vi "TDC_main.vi"() -> ()   [LabVIEW 2014]
panel:
  out "建过表":bool
  out "时间多道状态":string
  in  "放大":bool
  in  "复位":bool
  in  "是否需要建立修正表":bool
  out "时间谱":dbl[](array[numeric])
  out "修正后时间":dbl[](array[numeric])
  out "b查找表":dbl[](graph)
  out "a查找表":dbl[](graph)
  out "b积分表":dbl[](array[numeric])
  out "a积分表":dbl[](array[numeric])
  out "b码密度":dbl[](graph)
  out "a码密度":dbl[](graph)
  out "码密度数据量":dbl
  out "b细时间分布":dbl[](array[numeric])
  out "a细时间分布谱":dbl[](array[numeric])
  out "时间数据":u32[](array[numeric])
  out "起始时间":dbl
  in  "电压":u16=500
  in  "收发数据":T1(ring)
  out "保存灯":bool
  out "寻峰灯":bool
  out "状态灯":bool
  in  "按键检测":enum16{"空闲", "开始", "停止", "寻峰", "保存", "退出"}(ring)
  in  "保存":bool
  in  "寻峰":bool
  in  "停止":bool
  in  "开始":bool
  out "时间分布谱":dbl[](graph)
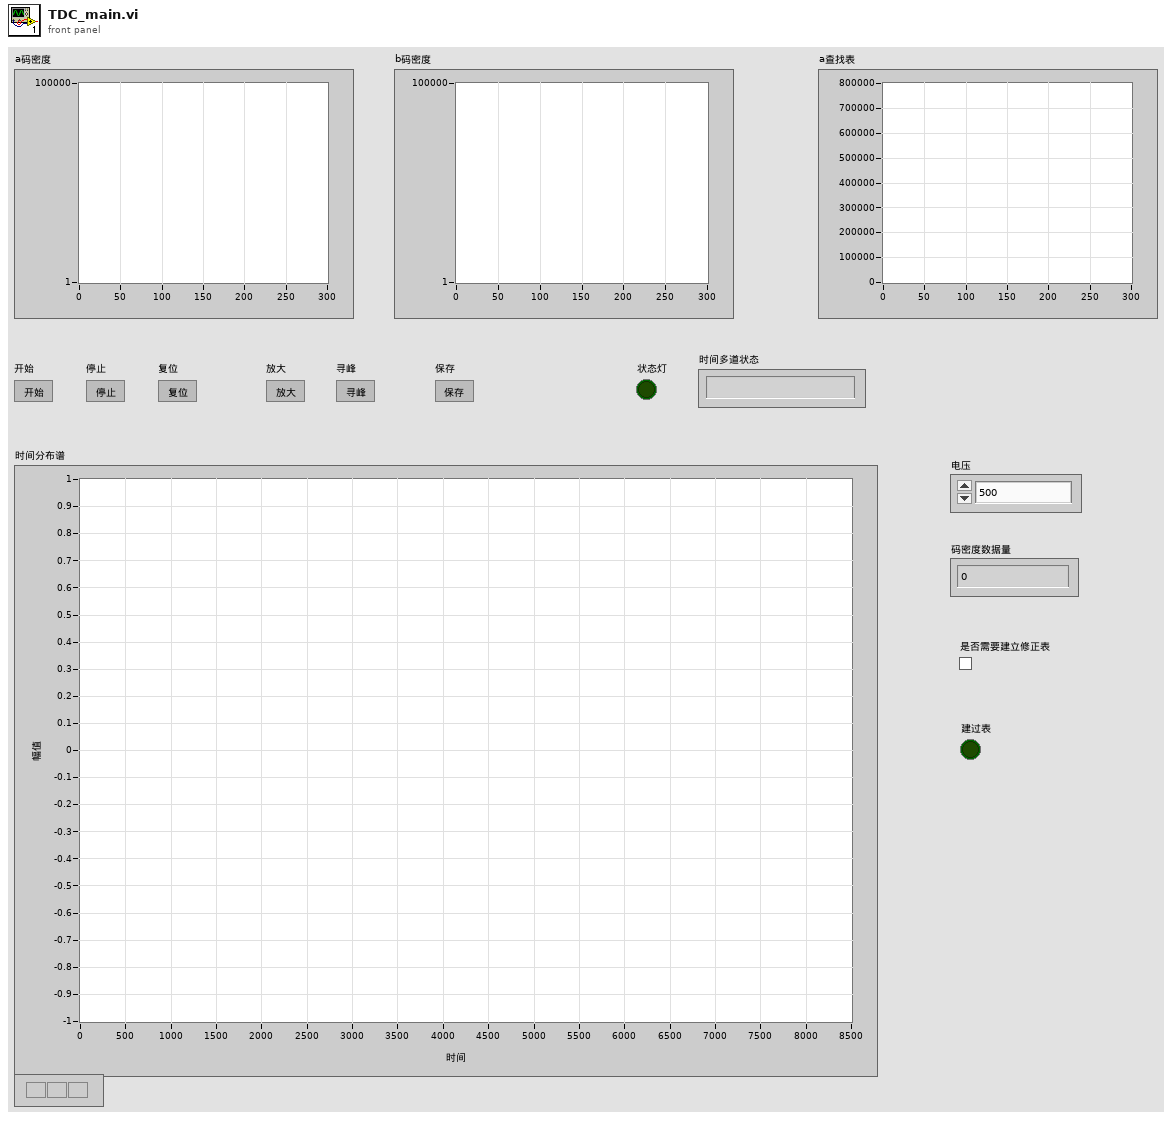
[diagram p1: front panel]
types:
  T1 = enum16{"空闲", "配置", "使能", "建立码密度表", "建立查找表", "显示时间谱"}
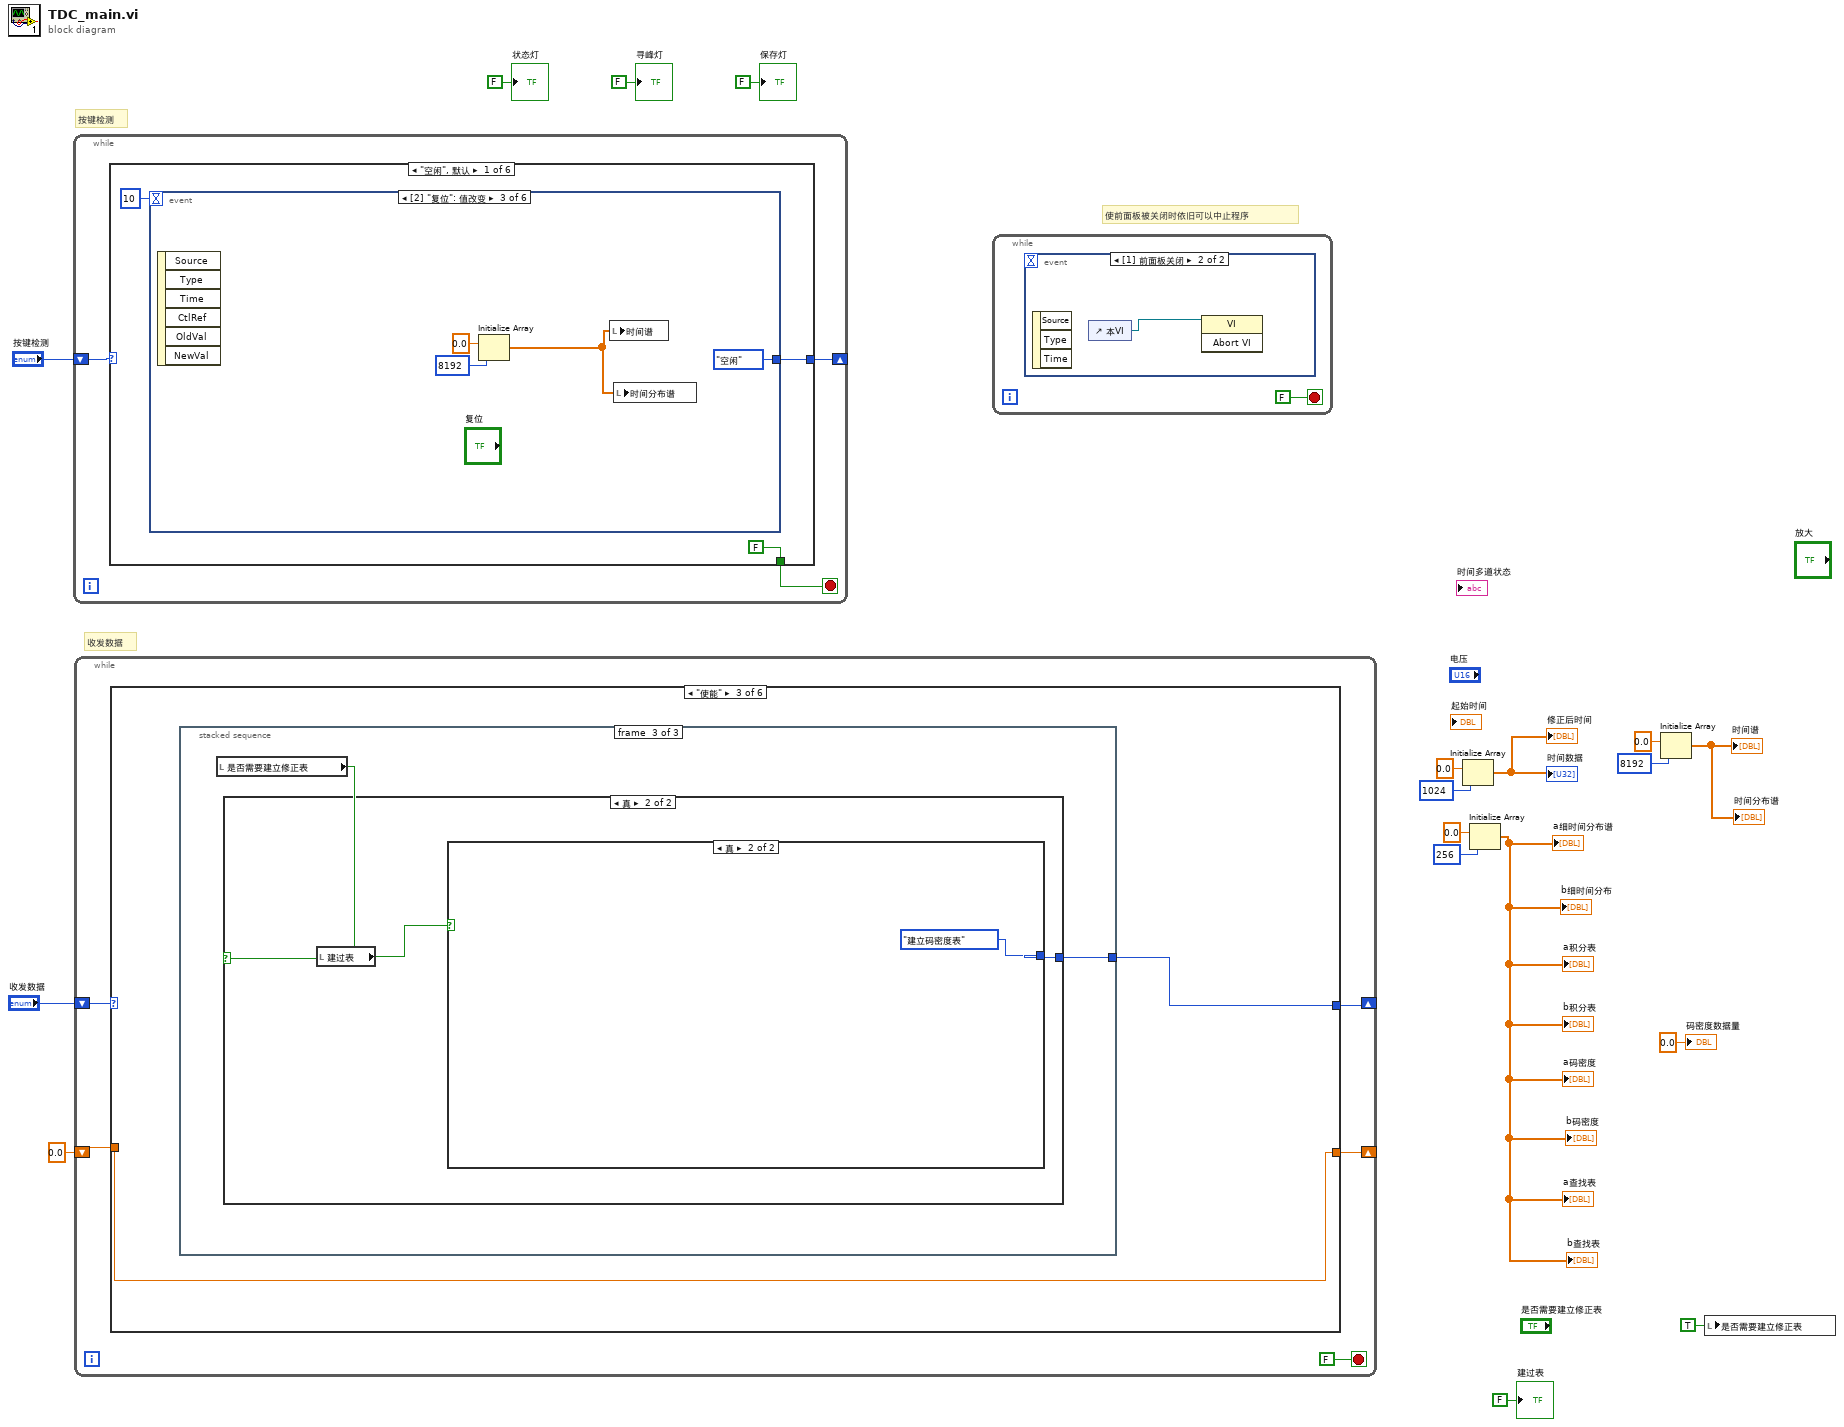
[diagram p0: block diagram]
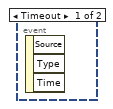
[diagram p2: hidden frame]
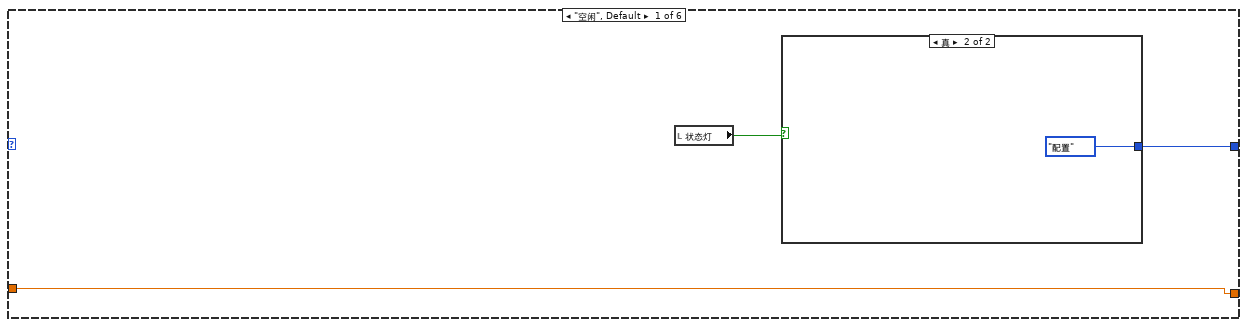
[diagram p3: hidden frame]
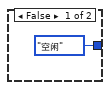
[diagram p4: hidden frame]
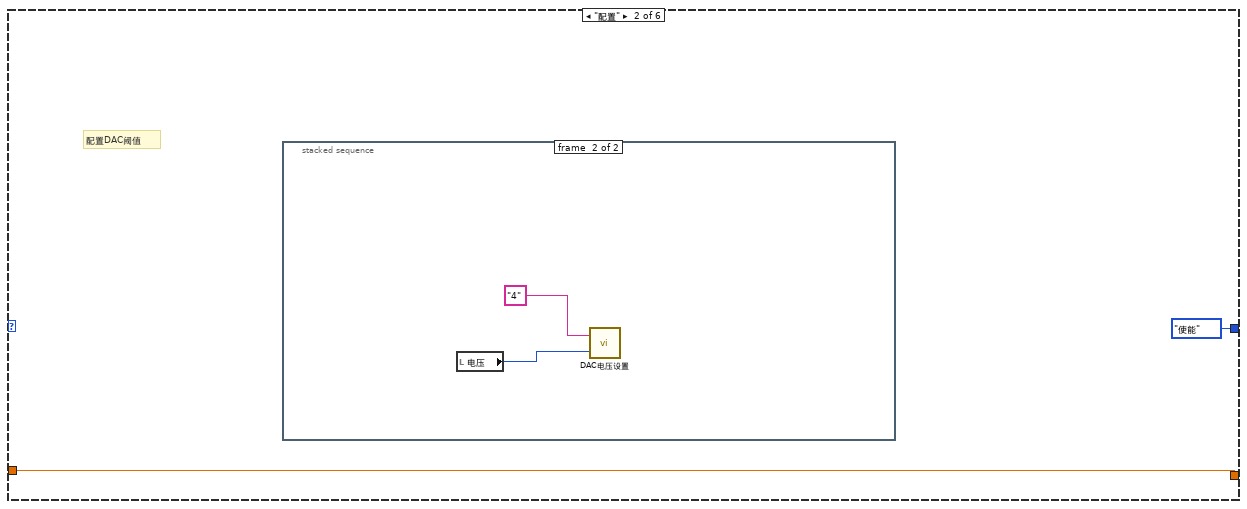
[diagram p5: hidden frame]
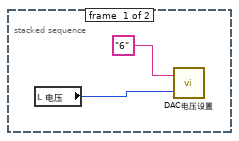
[diagram p6: hidden frame]
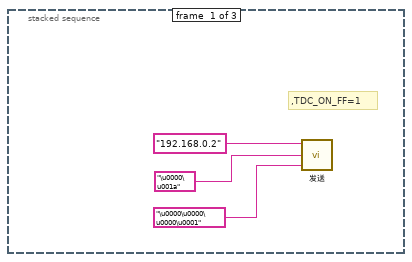
[diagram p7: hidden frame]
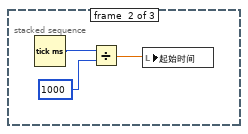
[diagram p8: hidden frame]
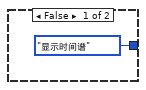
[diagram p9: hidden frame]
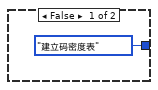
[diagram p10: hidden frame]
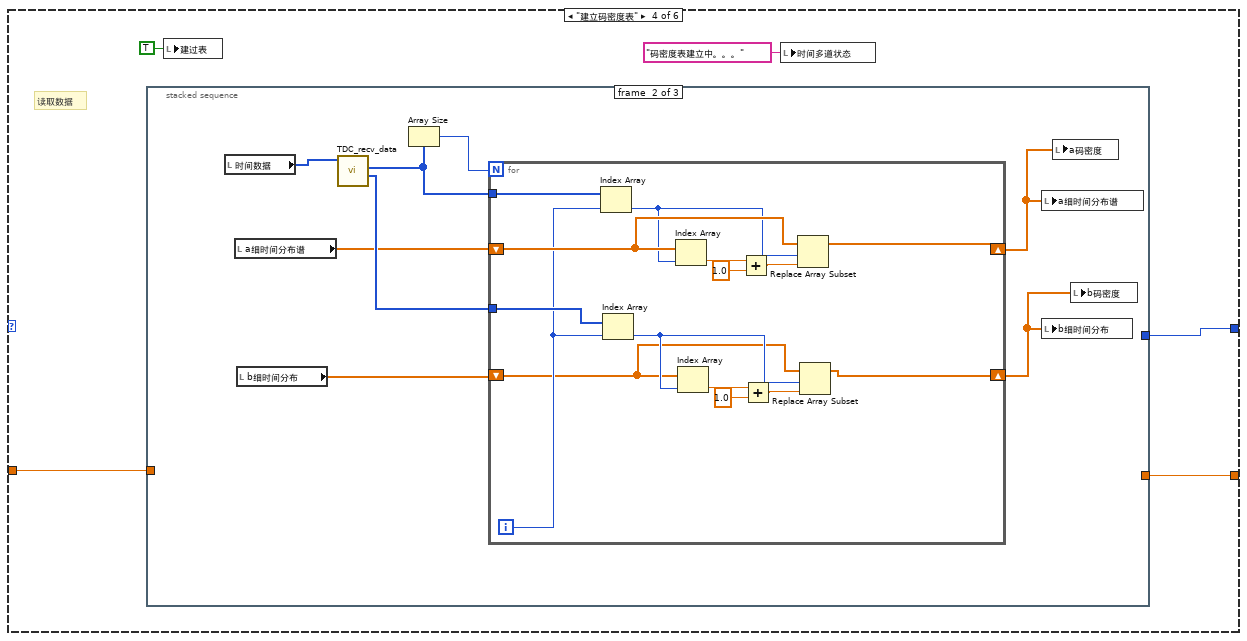
[diagram p11: hidden frame]
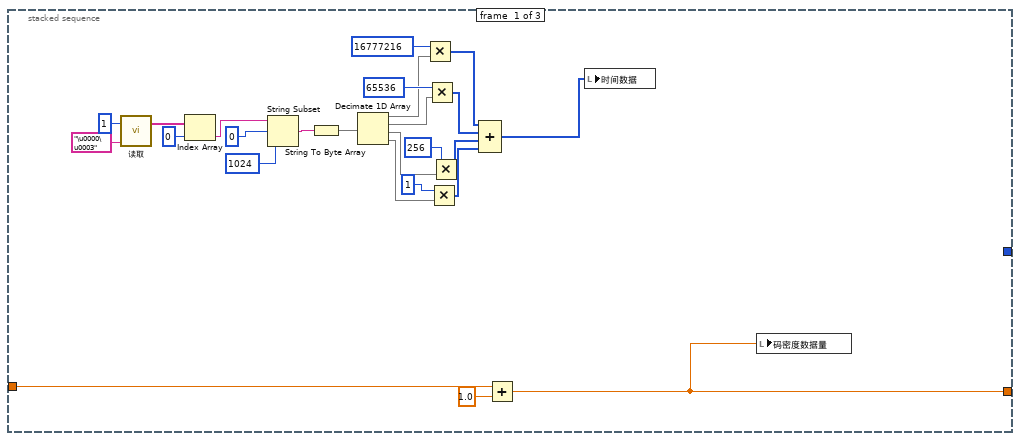
[diagram p12: hidden frame]
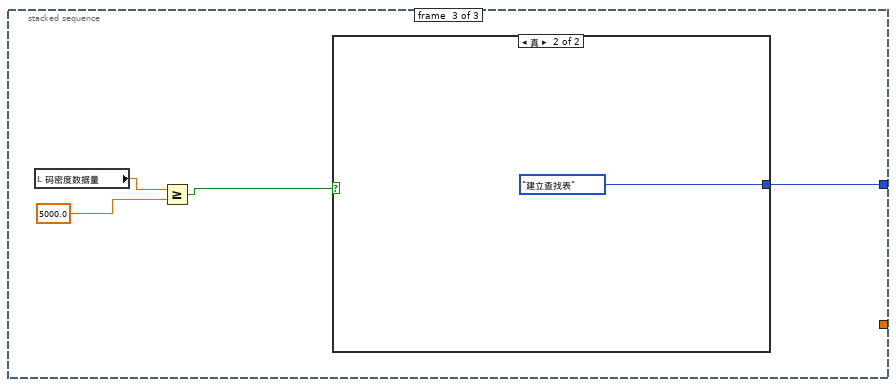
[diagram p13: hidden frame]
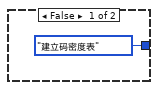
[diagram p14: hidden frame]
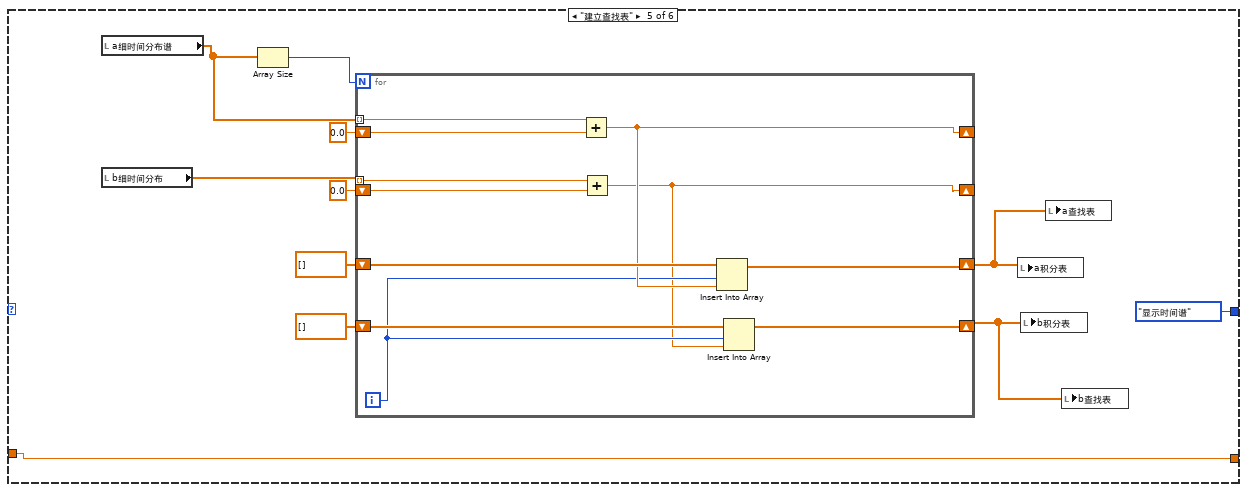
[diagram p15: hidden frame]
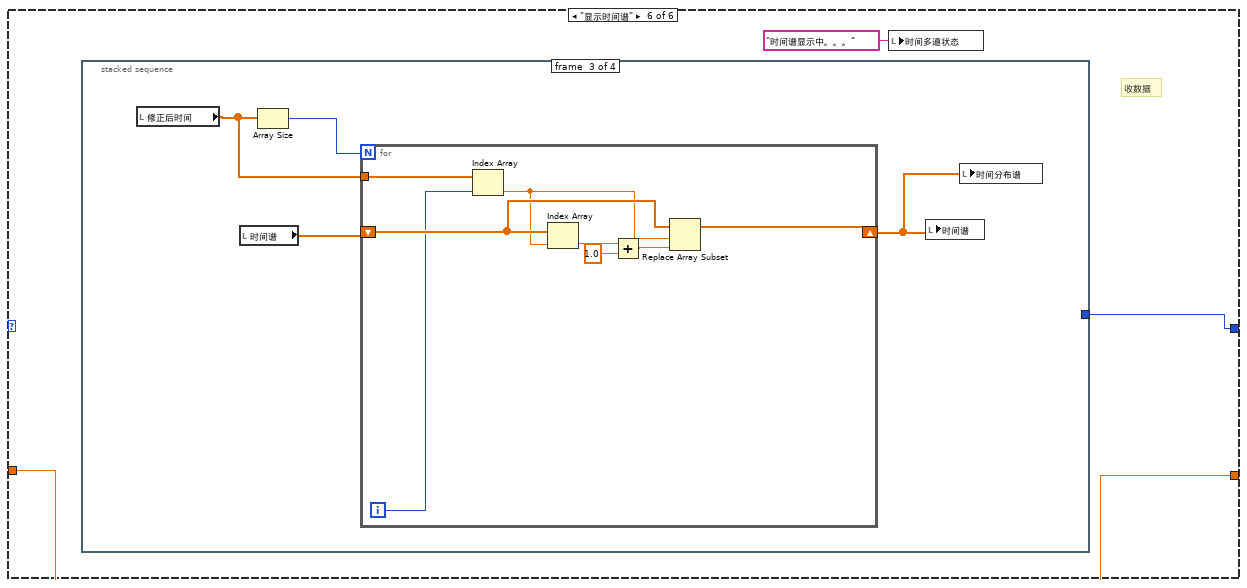
[diagram p16: hidden frame]
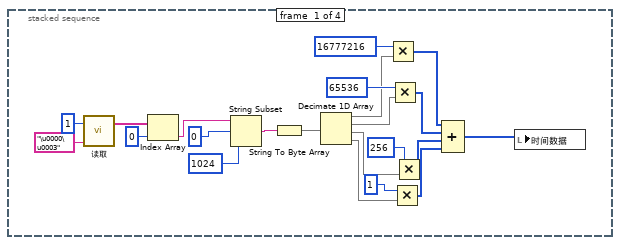
[diagram p17: hidden frame]
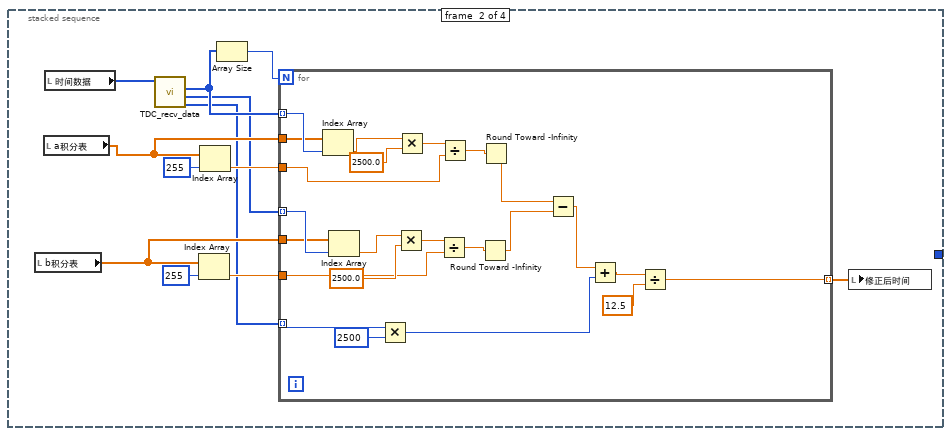
[diagram p18: hidden frame]
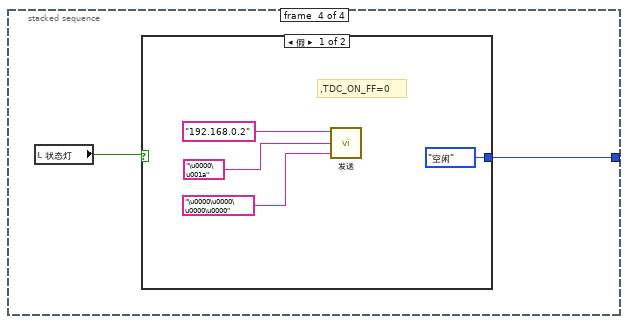
[diagram p19: hidden frame]
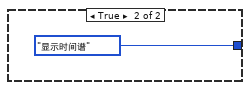
[diagram p20: hidden frame]
diagram:
  # "使前面板被关闭时依旧可以中止程序"
  # "收发数据"
  # "按键检测"
  n1 = while {
    shift-right: [w19] -> _
    shift-left: "按键检测" -> [w21]
    stop <- w20 stop-if-true
    n2 = case shown="\"空闲\", 默认" w21 {
      tunnel: [FALSE FALSE FALSE FALSE FALSE TRUE] -> w20
      tunnel: [w23 enum16{"空闲", "开始", "停止", "寻峰", "保存", "退出"}."空闲" ("按键检测") enum16{"空闲", "开始", "停止", "寻峰", "保存", "退出"}."空闲" ("按键检测") enum16{"空闲", "开始", "停止", "寻峰", "保存", "退出"}."空闲" ("按键检测") enum16{"空闲", "开始", "停止", "寻峰", "保存", "退出"}."空闲" ("按键检测") enum16{"空闲", "开始", "停止", "寻峰", "保存", "退出"}."空闲" ("按键检测")] -> w19
      frame "空闲", Default {
        n3 = event shown="[2] \"复位\": 值改变" {
          selector: _ -> [_ _ _ _ _ _]
          dyn-events: _ -> [_ _ _ _ _ _]
          timeout: 10 -> [_ _ _ _ _ _]
          tunnel: [enum16{"空闲", "开始", "停止", "寻峰", "保存", "退出"}."空闲" ("按键检测") enum16{"空闲", "开始", "停止", "寻峰", "保存", "退出"}."开始" ("按键检测") enum16{"空闲", "开始", "停止", "寻峰", "保存", "退出"}."空闲" ("按键检测") enum16{"空闲", "开始", "停止", "寻峰", "保存", "退出"}."停止" ("按键检测") enum16{"空闲", "开始", "停止", "寻峰", "保存", "退出"}."寻峰" ("按键检测") enum16{"空闲", "开始", "停止", "寻峰", "保存", "退出"}."保存" ("按键检测")] -> w23
          event Timeout {
            n4 = event-data() -> ()  [unwired: 1 in, 3 out]
          }
          event "开始": Value Change {
            n5 = event-data() -> ()  [unwired: 1 in, 6 out]
          }
          event "复位": Value Change {
            n6 = event-data() -> ()  [unwired: 1 in, 6 out]
            n7 = Initialize Array(0.0 ("元素"), 8192 ("维数大小")) -> (w27:dbl[])
            n8 = local write "时间谱"(w27) -> ()
            n9 = local write "时间分布谱"(w27) -> ()
          }
          event "停止": Value Change {
            n10 = event-data() -> ()  [unwired: 1 in, 6 out]
          }
          event "寻峰": Value Change {
            n11 = event-data() -> ()  [unwired: 1 in, 6 out]
          }
          event "保存": Value Change {
            n12 = event-data() -> ()  [unwired: 1 in, 6 out]
          }
        }
      }
      frame "开始" {
        n13 = local write "状态灯"(TRUE ("状态灯")) -> ()
      }
      frame "停止" {
        n14 = local write "状态灯"(FALSE ("状态灯")) -> ()
      }
      frame "寻峰" {
        n15 = local write "寻峰灯"(TRUE ("寻峰灯")) -> ()
      }
      frame "保存" {
        n16 = local write "保存灯"(TRUE ("保存灯")) -> ()
      }
      frame "退出" {
      }
    }
  }
  n17 = while {
    shift-right: [w50] -> _
    shift-left: "收发数据" -> [w52]
    shift-right: [w49] -> _
    shift-left: 0.0 -> [w48]
    stop <- FALSE stop-if-true
    n18 = case shown="\"使能\"" w52 {
      tunnel: [w54 T1."使能" ("收发数据") w64 w81 T1."显示时间谱" ("收发数据") w161] -> w50
      tunnel: [w53 w58 w65 w83 w148 w162] -> w49
      tunnel: w48 -> [w53 w58 w65 w82 w148 w162]
      frame "空闲", Default {
        n19 = local read "状态灯"() -> (w55:bool)
        n20 = case shown="真" w55 {
          tunnel: [T1."空闲" ("收发数据") T1."配置" ("收发数据")] -> w54
          frame False {
          }
          frame True {
          }
        }
      }
      frame "配置" {
        # "配置DAC阈值"
        n21 = stacked-sequence {
          frame #0 {
            n22 = local read "电压"() -> (w60:u16)
            n23 = call "DAC电压设置.vi"("电压"=w60, "cmd_channel(8bit)"="6") -> ()  [unwired: 1 in]
          }
          frame #1 {
            n24 = local read "电压"() -> (w62:u16)
            n25 = call "DAC电压设置.vi"("电压"=w62, "cmd_channel(8bit)"="4") -> ()  [unwired: 1 in]
          }
        }
      }
      frame "使能" {
        n26 = stacked-sequence {
          tunnel: [_ _ w73] -> w64
          frame #0 {
            # ",TDC_ON_FF=1"
            n27 = call "发送.vi"("数据（32bit）"="\u0000\u0000\u0000\u0001", "命令(16bit)"="\u0000\u001a", "目标IP"="192.168.0.2") -> ()  [unwired: 1 out]
          }
          frame #1 {
            n28 = Tick Count (ms)() -> (millisecond timer value=w69:u32)
            n29 = Divide(x=w69, y=u32 1000) -> (x/y=w71:dbl)
            n30 = local write "起始时间"(w71) -> ()
          }
          frame #2 {
            n31 = local read "是否需要建立修正表"() -> (w72:bool)
            n32 = case shown="真" w72 {
              tunnel: [T1."显示时间谱" ("收发数据") w76] -> w73
              frame False {
              }
              frame True {
                n33 = local read "建过表"() -> (w75:bool)
                n34 = case shown="真" w75 {
                  tunnel: [T1."建立码密度表" ("收发数据") T1."建立码密度表" ("收发数据")] -> w76
                  frame False {
                  }
                  frame True {
                  }
                }
              }
            }
          }
        }
      }
      frame "建立码密度表" {
        # "读取数据"
        n35 = stacked-sequence {
          tunnel: [w85 _ _] -> w83
          tunnel: w82 -> [w87 _ _]
          tunnel: [_ _ w132] -> w81
          frame #0 {
            n36 = call "读取.vi"("命令"="\u0000\u0003", "帧数"=1) -> ("数组"=w107:string[])  [unwired: 1 out]
            n37 = Index Array(array=w107, index=0 ("索引")) -> (element=w103:string)
            n38 = String Subset(string=w103, offset (0)=0 ("偏移量(0)"), length (rest)=1024 ("长度（剩余）")) -> (substring=w102:string)
            n39 = String To Byte Array(string=w102) -> (unsigned byte array=w101:u8[])
            n40 = Decimate 1D Array(w101) -> (w91:u8[], w92:u8[], w98:u8[], w97:u8[])
            n41 = Multiply(x=u32 16777216, y=w91) -> (x*y=w89:u32[])
            n42 = Multiply(x=u32 65536, y=w92) -> (x*y=w90:u32[])
            n43 = Multiply(x=u32 1, y=w97) -> (x*y=w95:u32[])
            n44 = Multiply(x=u32 256, y=w98) -> (x*y=w96:u32[])
            n45 = Compound Arithmetic op=ADD(w89, w90, w96, w95) -> (w88:u32[])
            n46 = Add(x=w87, y=1.0) -> (x+y=w85:dbl)
            n47 = local write "时间数据"(w88) -> ()
            n48 = local write "码密度数据量"(w85) -> ()
          }
          frame #1 {
            n49 = local read "时间数据"() -> (w116:u32[])
            n50 = local read "a细时间分布谱"() -> (w112:dbl[])
            n51 = local read "b细时间分布"() -> (w111:dbl[])
            n52 = call "TDC_recv_data.vi"("时间数据"=w116) -> ("b细计数"=w113:i32[], "a细计数"=w114:i32[])  [unwired: 1 out]
            n53 = Array Size(array=w114) -> (size(s)=w115:i32)
            n54 = for {
              N: w115 -> [_]
              tunnel: w114 -> [w131]
              tunnel: w113 -> [w122]
              shift-right: [w129] -> w110
              shift-left: w112 -> [w128]
              shift-right: [w119] -> w109
              shift-left: w111 -> [w120]
              i -> [w121]
              n55 = Index Array(array=w131, index=w121) -> (element=w127:i32)
              n56 = Index Array(array=w122, index=w121) -> (element=w124:i32)
              n57 = Index Array(array=w128, index=w127) -> (element=w130:dbl)
              n58 = Index Array(array=w120, index=w124) -> (element=w125:dbl)
              n59 = Add(x=w130, y=1.0) -> (x+y=w126:dbl)
              n60 = Add(x=w125, y=1.0) -> (x+y=w123:dbl)
              n61 = Replace Array Subset(array=w128, new element=w126, index=w127) -> (w129:dbl[])
              n62 = Replace Array Subset(array=w120, new element=w123, index=w124) -> (w119:dbl[])
            }
            n63 = local write "a细时间分布谱"(w110) -> ()
            n64 = local write "b细时间分布"(w109) -> ()
            n65 = local write "a码密度"(w110) -> ()
            n66 = local write "b码密度"(w109) -> ()
          }
          frame #2 {
            n67 = local read "码密度数据量"() -> (w135:dbl)
            n68 = Greater Or Equal?(x=w135, y=5000.0) -> (x >= y?=w133:bool)
            n69 = case shown="真" w133 {
              tunnel: [T1."建立码密度表" ("收发数据") T1."建立查找表" ("收发数据")] -> w132
              frame False {
              }
              frame True {
              }
            }
          }
        }
        n70 = local write "建过表"(TRUE ("建过表")) -> ()
        n71 = local write "时间多道状态"("码密度表建立中。。。" ("时间多道状态")) -> ()
      }
      frame "建立查找表" {
        n72 = local read "a细时间分布谱"() -> (w145:dbl[])
        n73 = local read "b细时间分布"() -> (w142:dbl[])
        n74 = Array Size(array=w145) -> (size(s)=w146:i32)
        n75 = for {
          N: w146 -> [_]
          tunnel: w145 -> [w159] mode=indexing
          shift-right: [w155] -> _
          shift-left: 0.0 -> [w158]
          shift-right: [w156] -> w139
          shift-left: dbl[] [] -> [w157]
          tunnel: w142 -> [w154] mode=indexing
          shift-right: [w150] -> _
          shift-left: 0.0 -> [w153]
          shift-right: [w149] -> w138
          shift-left: dbl[] [] -> [w152]
          i -> [w151]
          n76 = Add(x=w159, y=w158) -> (x+y=w155:dbl)
          n77 = Add(x=w154, y=w153) -> (x+y=w150:dbl)
          n78 = Insert Into Array(array=w157, index=w151, new element=w155) -> (w156:dbl[])
          n79 = Insert Into Array(array=w152, index=w151, new element=w150) -> (w149:dbl[])
        }
        n80 = local write "a积分表"(w139) -> ()
        n81 = local write "b积分表"(w138) -> ()
        n82 = local write "a查找表"(w139) -> ()
        n83 = local write "b查找表"(w138) -> ()
      }
      frame "显示时间谱" {
        # "收数据"
        n84 = stacked-sequence {
          tunnel: [_ _ _ w232] -> w161
          frame #0 {
            n85 = call "读取.vi"("命令"="\u0000\u0003", "帧数"=1) -> ("数组"=w183:string[])  [unwired: 1 out]
            n86 = Index Array(array=w183, index=0 ("索引")) -> (element=w179:string)
            n87 = String Subset(string=w179, offset (0)=0 ("偏移量(0)"), length (rest)=1024 ("长度（剩余）")) -> (substring=w178:string)
            n88 = String To Byte Array(string=w178) -> (unsigned byte array=w177:u8[])
            n89 = Decimate 1D Array(w177) -> (w167:u8[], w168:u8[], w174:u8[], w173:u8[])
            n90 = Multiply(x=u32 16777216, y=w167) -> (x*y=w165:u32[])
            n91 = Multiply(x=u32 65536, y=w168) -> (x*y=w166:u32[])
            n92 = Multiply(x=u32 1, y=w173) -> (x*y=w171:u32[])
            n93 = Multiply(x=u32 256, y=w174) -> (x*y=w172:u32[])
            n94 = Compound Arithmetic op=ADD(w165, w166, w172, w171) -> (w163:u32[])
            n95 = local write "时间数据"(w163) -> ()
          }
          frame #1 {
            n96 = local read "b积分表"() -> (w188:dbl[])
            n97 = local read "a积分表"() -> (w192:dbl[])
            n98 = local read "时间数据"() -> (w196:u32[])
            n99 = call "TDC_recv_data.vi"("时间数据"=w196) -> ("粗计数"=w186:i32[], "b细计数"=w190:i32[], "a细计数"=w193:i32[])
            n100 = Index Array(array=w188, index=255 ("索引")) -> (element=w187:dbl)
            n101 = Index Array(array=w192, index=255 ("索引")) -> (element=w191:dbl)
            n102 = Array Size(array=w193) -> (size(s)=w195:i32)
            n103 = for {
              N: w195 -> [_]
              tunnel: w193 -> [w219] mode=indexing
              tunnel: w192 -> [w218]
              tunnel: w191 -> [w214]
              tunnel: w190 -> [w212] mode=indexing
              tunnel: w188 -> [w211]
              tunnel: w187 -> [w206]
              tunnel: w186 -> [w205] mode=indexing
              tunnel: [w197] -> w185 mode=indexing
              n104 = Index Array(array=w218, index=w219) -> (element=w217:dbl)
              n105 = Index Array(array=w211, index=w212) -> (element=w207:dbl)
              n106 = Multiply(x=w205, y=2500) -> (x*y=w201:i32)
              n107 = Multiply(x=w207, y=2500.0) -> (x*y=w209:dbl)
              n108 = Multiply(x=w217, y=2500.0) -> (x*y=w215:dbl)
              n109 = Divide(x=w209, y=w206) -> (x/y=w208:dbl)
              n110 = Divide(x=w215, y=w214) -> (x/y=w213:dbl)
              n111 = Round Toward -Infinity(1:w208) -> (0:w202:dbl)
              n112 = Round Toward -Infinity(1:w213) -> (0:w203:dbl)
              n113 = Subtract(x=w203, y=w202) -> (x-y=w200:dbl)
              n114 = Add(x=w200, y=w201) -> (x+y=w199:dbl)
              n115 = Divide(x=w199, y=12.5) -> (x/y=w197:dbl)
            }
            n116 = local write "修正后时间"(w185) -> ()
          }
          frame #2 {
            n117 = local read "修正后时间"() -> (w222:dbl[])
            n118 = local read "时间谱"() -> (w221:dbl[])
            n119 = Array Size(array=w222) -> (size(s)=w223:i32)
            n120 = for {
              N: w223 -> [_]
              tunnel: w222 -> [w231]
              shift-right: [w229] -> w220
              shift-left: w221 -> [w228]
              i -> [w225]
              n121 = Index Array(array=w231, index=w225) -> (element=w227:dbl)
              n122 = Index Array(array=w228, index=w227) -> (element=w230:dbl)
              n123 = Add(x=w230, y=1.0) -> (x+y=w226:dbl)
              n124 = Replace Array Subset(array=w228, new element=w226, index=w227) -> (w229:dbl[])
            }
            n125 = local write "时间谱"(w220) -> ()
            n126 = local write "时间分布谱"(w220) -> ()
          }
          frame #3 {
            n127 = local read "状态灯"() -> (w233:bool)
            n128 = case shown="假" w233 {
              tunnel: [T1."空闲" ("收发数据") T1."显示时间谱" ("收发数据")] -> w232
              frame False {
                # ",TDC_ON_FF=0"
                n129 = call "发送.vi"("数据（32bit）"="\u0000\u0000\u0000\u0000", "命令(16bit)"="\u0000\u001a", "目标IP"="192.168.0.2") -> ()  [unwired: 1 out]
              }
              frame True {
              }
            }
          }
        }
        n130 = local write "时间多道状态"("时间谱显示中。。。" ("时间多道状态")) -> ()
      }
    }
  }
  n131 = while {
    stop <- FALSE stop-if-true
    n132 = event shown="[1] 前面板关闭" {
      selector: _ -> [_ _]
      dyn-events: _ -> [_ _]
      timeout: _ -> [_ _]
      event Timeout {
        n133 = event-data() -> ()  [unwired: 1 in, 3 out]
      }
      event Panel Close {
        n134 = event-data() -> ()  [unwired: 1 in, 3 out]
        n135 = control-ref of="本VI"() -> (w240:refnum<vi>)
        n136 = invoke class="VI" method="Abort VI"(reference=w240) -> ()  [unwired: 2 in, 3 out]
      }
    }
  }
  n137 = Initialize Array(0.0 ("元素"), 1024 ("维数大小")) -> (→"时间数据" →"修正后时间":dbl[])
  n138 = Initialize Array(0.0 ("元素"), 256 ("维数大小")) -> (→"a细时间分布谱" →"b细时间分布" →"a积分表" →"b积分表" →"a码密度" →"b码密度" →"a查找表" →"b查找表":dbl[])
  n139 = Initialize Array(0.0 ("元素"), 8192 ("维数大小")) -> (→"时间谱" →"时间分布谱":dbl[])
  n140 = local write "是否需要建立修正表"(TRUE ("是否需要建立修正表")) -> ()
  "状态灯" <- FALSE ("状态灯")
  "寻峰灯" <- FALSE ("寻峰灯")
  "保存灯" <- FALSE ("保存灯")
  "码密度数据量" <- 0.0 ("码密度数据量")
  "建过表" <- FALSE ("建过表")
